vi "GCMPlugin_IsSupportingItem.vi"(8 "error in (no error)":errorcluster, 9 "VI Reference":refnum<vi>, 10 "ProjectItem Refnum":refnum<vi>, 11 "_BasicClassDocumentation in":refnum<class "BasicClassDocumentation.lvclass">) -> (0 "error out":errorcluster, 2 "IsSupportingItem":bool, 3 "_BasicClassDocumentation out":refnum<class "BasicClassDocumentation.lvclass">)   [LabVIEW 2014, in "BasicClassDocumentation.lvlib" / "BasicClassDocumentation.lvclass"]
uses:
  BasicClassDocumentation.lvclass
  Utilites/_ProjectItemsUtilities/_ProjectItemsUtilities.lvlib
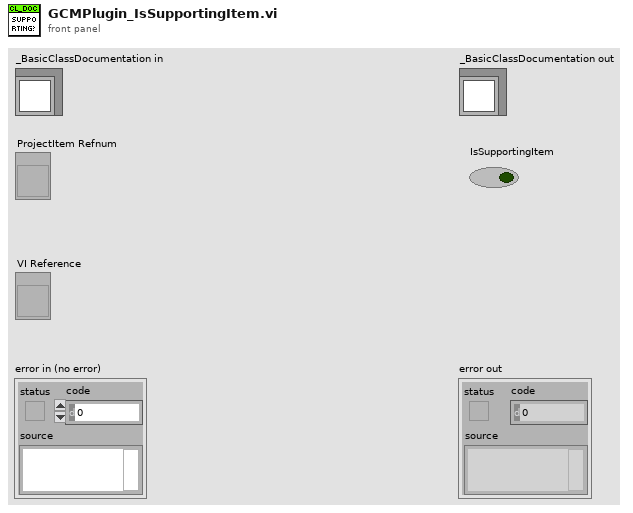
[diagram p1: front panel]
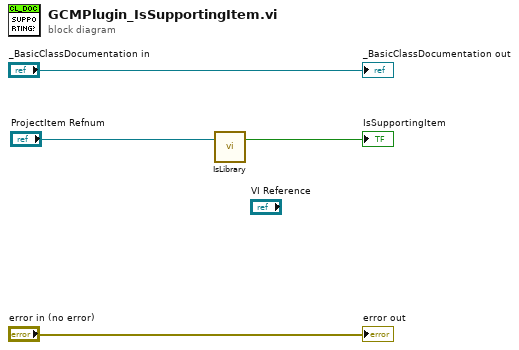
[diagram p0: block diagram]
diagram:
  n1 = call "IsLibrary.vi"("ProjectItem Refnum"="ProjectItem Refnum") -> ("IsLibrary?"=→"IsSupportingItem":bool)  [unwired: 2 in]
  "error out" <- "error in (no error)"
  "_BasicClassDocumentation out" <- "_BasicClassDocumentation in"
